vi "drivetrainSelector.vi"(6 "AutoTrackButton":bool, 8 "rearRight":dbl, 9 "rearLeft":dbl, 10 "frontRight":dbl, 11 "frontLeft":dbl) -> ()   [LabVIEW 2011]
panel:
  in  "CameraXPosition":dbl
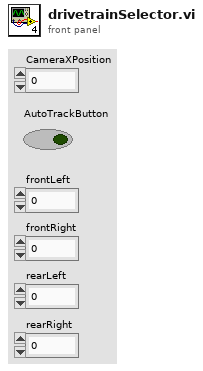
[diagram p1: front panel]
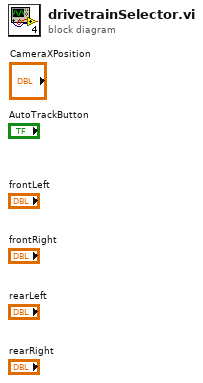
[diagram p0: block diagram]
diagram:
